vi "HelloWorld.vi"() -> ()   [LabVIEW 2012]
uses:
  <vilib>/rvi/eio/common/nirviEmuTemplateMethod_errors.vi
  <vilib>/eio/EIONode/EIONode.xnode
panel:
  in  "stop":bool
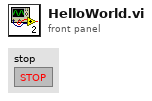
[diagram p1: front panel]
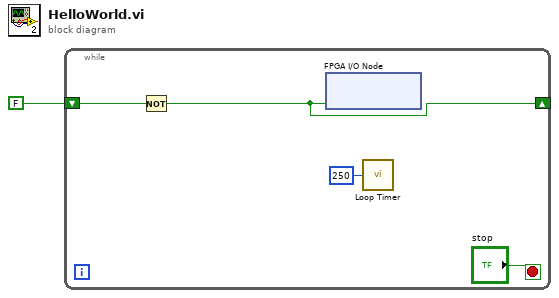
[diagram p0: block diagram]
diagram:
  n1 = while {
    shift-right: [w3] -> _
    shift-left: FALSE -> [w4]
    stop <- "stop" stop-if-true
    n2 = Not(x=w4) -> (.not. x?=w3:bool)
    n3 = xnode "FPGA I/O Node"("FPGA LED"=w3) -> ()  [unwired: 1 in, 1 out]
    n4 = call "Loop Timer"("Count(Ticks)"=u32 250) -> ()  [unwired: 1 out]
  }
